vi "buffer_template.vi"(8 "error in":errorcluster, 11 "handle":i32) -> (0 "error out":errorcluster, 3 "buf out":string)   [LabVIEW 2020]
uses:
  client/client.lvlib
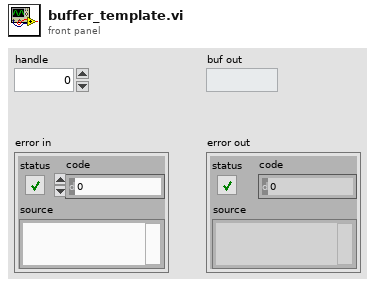
[diagram p1: front panel]
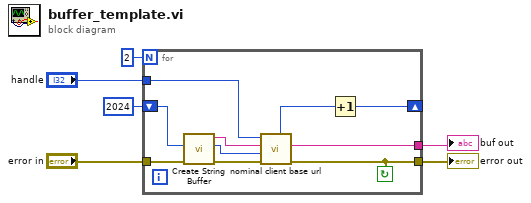
[diagram p0: block diagram]
diagram:
  n1 = for {
    N: 2 -> [_]
    tunnel: "handle" -> [w16]
    tunnel: [w15] -> w1
    shift-right: [w7] -> _
    shift-left: 2024 ("Buffer Size (1024)") -> [w12]
    tunnel: "error in" -> [w10]
    tunnel: [w8] -> w3
    stop <- w8 continue-if-true
    n2 = call "Create String Buffer.vi"("error in"=w10, "Buffer Size (1024)"=w12) -> ("error out"=w11:errorcluster, "dub Buffer Size"=w13:i32, "String Buffer"=w14:string)  [unwired: 7 in]
    n3 = call "nominal client base url.vi"("error in (no error)"=w11, "cap"=w13, "buf"=w14, "client"=w16) -> ("error out"=w8:errorcluster, "buf out"=w15:string, "out_needed out"=w9:u32)  [unwired: 4 in, 1 out]
    n4 = Increment(x=w9) -> (x+1=w7:u32)
  }
  "error out" <- w3
  "buf out" <- w1
